vi "Clean Up References.vi"(8 "error in (no error)":errorcluster, 11 "Subpanel.Edit in":refnum<class "Subpanel.Edit.lvclass">) -> (0 "error out":errorcluster, 3 "Subpanel.Edit out":refnum<class "Subpanel.Edit.lvclass">)   [LabVIEW 2019, in "Subpanel.Edit.lvclass"]
uses:
  Subpanel.Edit.lvclass
  Subpanel.Edit.lvclass/Subpanel.Edit.ctl
  Edit/Edit/Edit.lvclass
  C:/Program Files (x86)/National Instruments/LabVIEW 2019/vi.lib/JKI/JKI SMO/SMO/SMO.lvclass
  <vilib>/JKI/JKI SMO/SMO/SMO.lvclass
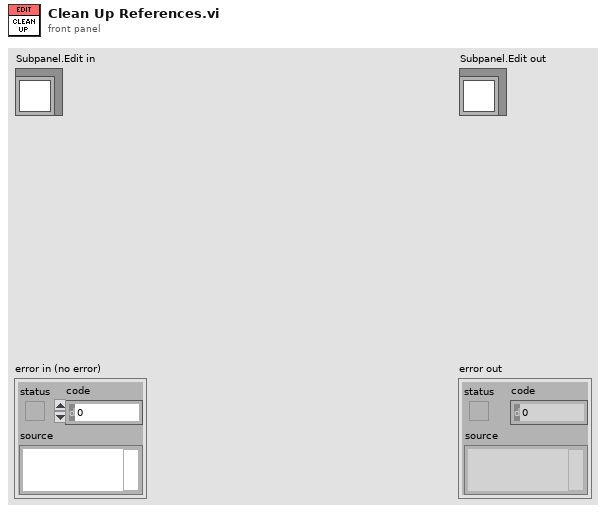
[diagram p1: front panel]
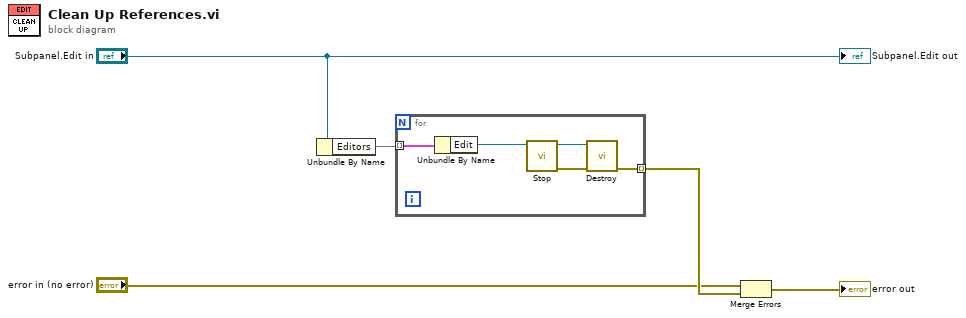
[diagram p0: block diagram]
diagram:
  n1 = Unbundle By Name("Subpanel.Edit in") -> ("Editors"=w5:map{string, refnum<class "Edit.lvclass">})
  n2 = for {
    tunnel: w5 -> [w10] mode=indexing
    tunnel: [w6] -> w3 mode=indexing
    n3 = Unbundle By Name(w10) -> ("Edit"=w9:refnum<class "Edit.lvclass">)
    n4 = call <vilib>:"Stop.vi"("SMO"=w9) -> ("error out"=w7:errorcluster, "SMO out"=w8:refnum<class "Edit.lvclass">)  [unwired: 9 in]
    n5 = call <vilib>:"Destroy.vi"("error in (no error)"=w7, "SMO"=w8) -> ("error out"=w6:errorcluster)  [unwired: 9 in]
  }
  n6 = Merge Errors("error in (no error)", w3) -> (→"error out":errorcluster)
  "Subpanel.Edit out" <- "Subpanel.Edit in"
